vi "CHlist Drag Start Event.vi"(8 "error in":errorcluster, 10 "Coords":T2, 11 "TreeControl in":refnum<vi>) -> (0 "error out":errorcluster, 3 "data":T1(array[cluster]))   [LabVIEW 2016]
uses:
  <vilib>/Utility/miscctls.llb/LVPoint32TypeDef.ctl
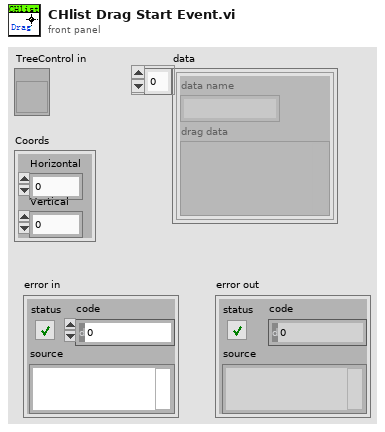
[diagram p1: front panel]
types:
  T1 = cluster{"data name":string, "drag data":variant}[]
  T2 = typedef "LVPoint32TypeDef.ctl" = cluster{"Horizontal":i32, "Vertical":i32}
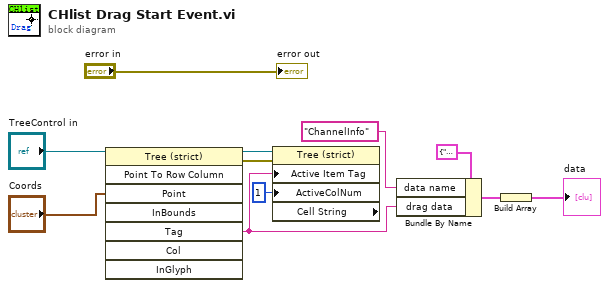
[diagram p0: block diagram]
diagram:
  n1 = invoke class="Tree (strict)" method="Point To Row Column"(reference="TreeControl in", "Point"="Coords") -> (reference out=w8:refnum<vi>, error out=w9:errorcluster, "Tag"=w11:string)  [unwired: 6 in, 5 out]
  n2 = property class="Tree (strict)" props=["Active Item Tag", "ActiveColNum", "Cell String"](reference=w8, error in=w9, "Active Item Tag"=w11, "ActiveColNum"=1 ("活动单元格:活动列数")) -> ()  [unwired: 3 out]
  n3 = Bundle By Name(cluster=cluster{"data name":string, "drag data":variant} {"data name"="", "drag data"=variant}, "data name"="ChannelInfo", "drag data"=w11) -> (w5:cluster{"data name":string, "drag data":variant})
  n4 = Build Array(w5) -> (→"data":T1)
  "error out" <- "error in"
